vi "MPUSBClose.vi"(8 "error in (no error)":errorcluster, 11 "handle":u32 format="%x") -> (0 "error out":errorcluster, 3 "return type":i32)   [LabVIEW 2019]
doc: "// MPUSBClose : closes a given handle.\n//\n// Note that \"input\" and \"output\" refer to the parameter designations in calls\n// to this function, which are the opposite of common sense from the\n// perspective of an application making the calls.\n\nWritten by: Complete Automated Solutions\nwww.CompleteAutomatedSolutions.com"
uses:
  mpusbapi.dll
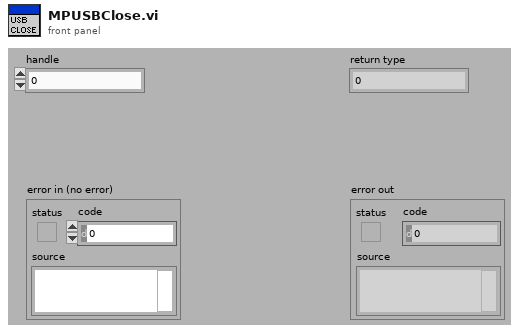
[diagram p1: front panel]
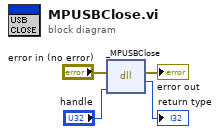
[diagram p0: block diagram]
diagram:
  n1 = dll-call lib="C:/Users/z003r4zd/Desktop/Point Contact Mods 2019/Automation/Actuonix/LAC+Labview+Example/Actuonix_LAC_LabVIEW_Example/USB_VIs/mpusbapi.dll" fn="_MPUSBClose"(error in="error in (no error)", "handle"="handle") -> (error out=→"error out":errorcluster, "return type"=→"return type":i32)  [unwired: 3 in, 1 out]
